vi "Stack completion.vi"() -> ()   [LabVIEW 2012]
panel:
  out "error out":errorcluster
  out "appended path":path
  in  "error in":errorcluster
  in  "Step":u32
  in  "Stop":u32
  in  "Start":u32
  in  "Stack folder":path
  in  "Fixed string portion":string
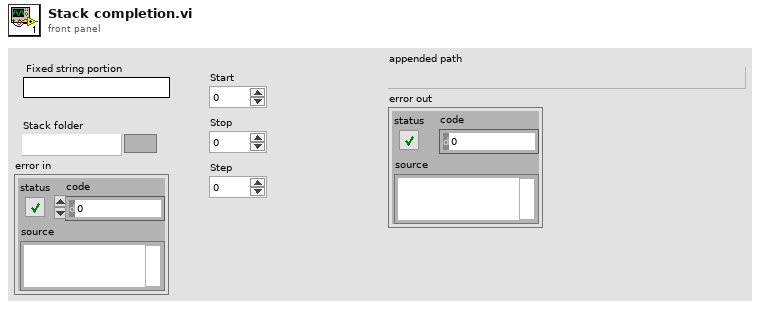
[diagram p1: front panel]
types:
  T1 = typedef "Image Type" = u32
  T2 = typedef "IMAQ Image.ctl" = refnum<image>
  T3 = cluster{"Rows Per Strip":i32, "Photometric":i32, "Compression Type":i32}
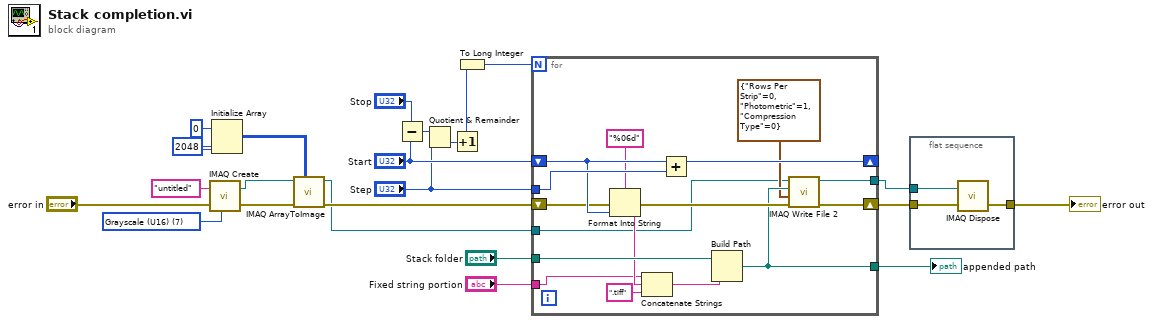
[diagram p0: block diagram]
diagram:
  w9 = T1 7 items=["Grayscale (U8)", "Grayscale (I16)", "Grayscale (SGL)", "Complex (CSG)", "RGB (U32)", "HSL (U32)", "RGB (U64)", "Grayscale (U16)"] ("Image Type")
  w22 = 2048 ("dimension size")
  n1 = call "IMAQ Create"("Image Name"="untitled", "Image Type"=w9, "error in (no error)"="error in") -> ("New Image"=w8:T2, "error out"=w7:errorcluster)  [unwired: 2 in]
  n2 = Initialize Array(u16 0 ("element"), w22, w22) -> (w6:u16[][])
  n3 = call "IMAQ ArrayToImage"("Image Pixels (U16)"=w6, "error in (no error)"=w7, "Image"=w8) -> ("error out"=w5:errorcluster, "Image Out"=w4:T2)  [unwired: 7 in]
  n4 = Subtract(x="Stop", y="Start") -> (x-y=w18:u32)
  n5 = Quotient & Remainder(x=w18, y="Step") -> (floor(x/y)=w17:u32)  [unwired: 1 out]
  n6 = Increment(x=w17) -> (x+1=w16:u32)
  n7 = To Long Integer(number=w16) -> (32bit integer=w15:i32)
  n8 = for {
    N: w15 -> [_]
    tunnel: "Stack folder" -> [w33]
    tunnel: "Fixed string portion" -> [w30]
    shift-right: [w36] -> _
    shift-left: "Start" -> [w37]
    tunnel: "Step" -> [w38]
    shift-right: [w27] -> w3
    shift-left: w5 -> [w35]
    tunnel: [w26] -> w12
    tunnel: w4 -> [w24]
    tunnel: [w24] -> w1
    n9 = Format Into String(format string="%06d", error in=w35, w37) -> (resulting string=w31:string, error out=w28:errorcluster)  [unwired: 1 in]
    n10 = Concatenate Strings(w30, w31, ".tiff" ("string")) -> (w32:string)
    n11 = Add(x=w37, y=w38) -> (x+y=w36:u32)
    n12 = Build Path(base path=w33, name or relative path=w32) -> (appended path=w26:path)
    n13 = call-poly "IMAQ Write File 2"("error in (no error)"=w28, "TIFF Options"=T3 {"Rows Per Strip"=0, "Photometric"=1, "Compression Type"=0}, "File Path"=w26, "Image"=w24) -> ("error out"=w27:errorcluster)  [unwired: 6 in, 1 out]
  }
  "appended path" <- w12
  n14 = flat-sequence {
    tunnel: w3 -> [w41]
    tunnel: [w40] -> w2
    tunnel: w1 -> [w39]
    frame #0 {
      n15 = call "IMAQ Dispose"("Image"=w39, "error in (no error)"=w41) -> ("error out"=w40:errorcluster)  [unwired: 4 in]
    }
  }
  "error out" <- w2
